vi "Add Expression.vi"(8 "error in (no error)":errorcluster, 9 "Section":enum16{"Main", "Setup", "Cleanup"}(ring), 10 "Expression":string, 11 "RT Sequence Ref in":refnum<k24>) -> (0 "error out":errorcluster, 3 "RT Sequence Ref out":refnum<k24>)   [LabVIEW 2016, in "RT Sequence Creator API.lvlib"]
uses:
  RT Sequence Creator API.lvlib
  NationalInstruments.VeriStand.RealTimeSequenceDefinitionApi
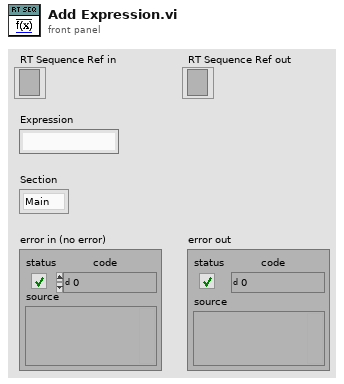
[diagram p1: front panel]
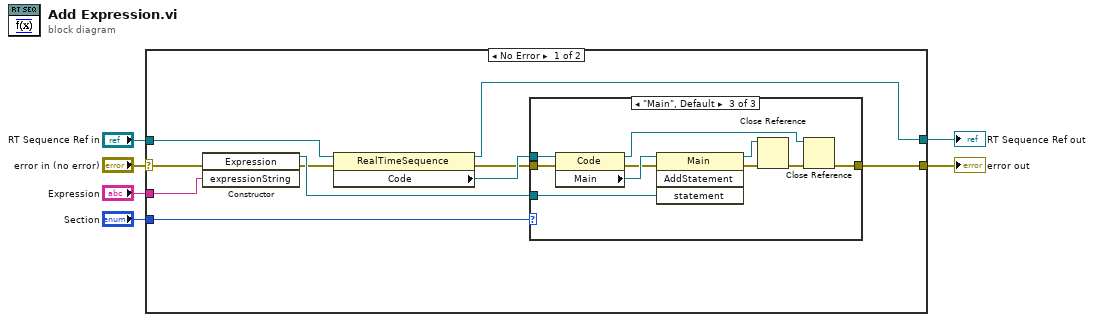
[diagram p0: block diagram]
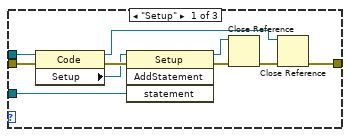
[diagram p2: hidden frame]
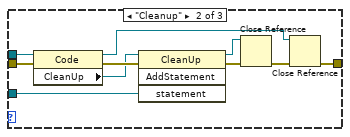
[diagram p3: hidden frame]
diagram:
  n1 = case shown="No Error" "error in (no error)" {
    selector: "error in (no error)" -> [w9 w47]
    tunnel: "RT Sequence Ref in" -> [w16 w48]
    tunnel: [w12 w47] -> w4
    tunnel: [w11 w48] -> w3
    tunnel: "Section" -> [w13 _]
    tunnel: "Expression" -> [w7 _]
    frame No Error {
      n2 = constructor class="Expression"(error in=w9, "expressionString"=w7) -> (reference out=w10:refnum<k24>, error out=w8:errorcluster)  [unwired: 2 in, 2 out]
      n3 = property class="RealTimeSequence"(reference=w16, error in=w8) -> (reference out=w11:refnum<k24>, error out=w14:errorcluster, "Code"=w15:refnum<k24>)
      n4 = case shown="\"Main\", Default" w13 {
        tunnel: w15 -> [w26 w36 w46]
        tunnel: w14 -> [w25 w35 w45]
        tunnel: [w20 w30 w38] -> w12
        tunnel: w10 -> [w17 w27 w37]
        frame "Setup" {
          n5 = property class="Code"(reference=w26, error in=w25) -> (reference out=w18:refnum<k24>, error out=w24:errorcluster, "Setup"=w23:refnum<k24>)
          n6 = invoke class="Setup" method="AddStatement"(reference=w23, error in=w24, "statement"=w17) -> (reference out=w19:refnum<k24>, error out=w22:errorcluster)  [unwired: 1 in, 2 out]
          n7 = Close Reference(reference=w19, error in (no error)=w22) -> (error out=w21:errorcluster)
          n8 = Close Reference(reference=w18, error in (no error)=w21) -> (error out=w20:errorcluster)
        }
        frame "Cleanup" {
          n9 = property class="Code"(reference=w36, error in=w35) -> (reference out=w28:refnum<k24>, error out=w31:errorcluster, "CleanUp"=w29:refnum<k24>)
          n10 = invoke class="CleanUp" method="AddStatement"(reference=w29, error in=w31, "statement"=w27) -> (reference out=w34:refnum<k24>, error out=w32:errorcluster)  [unwired: 1 in, 2 out]
          n11 = Close Reference(reference=w34, error in (no error)=w32) -> (error out=w33:errorcluster)
          n12 = Close Reference(reference=w28, error in (no error)=w33) -> (error out=w30:errorcluster)
        }
        frame "Main", Default {
          n13 = property class="Code"(reference=w46, error in=w45) -> (reference out=w39:refnum<k24>, error out=w43:errorcluster, "Main"=w44:refnum<k24>)
          n14 = invoke class="Main" method="AddStatement"(reference=w44, error in=w43, "statement"=w37) -> (reference out=w40:refnum<k24>, error out=w42:errorcluster)  [unwired: 1 in, 2 out]
          n15 = Close Reference(reference=w40, error in (no error)=w42) -> (error out=w41:errorcluster)
          n16 = Close Reference(reference=w39, error in (no error)=w41) -> (error out=w38:errorcluster)
        }
      }
    }
    frame Error {
    }
  }
  "RT Sequence Ref out" <- w3
  "error out" <- w4
